vi "Main.vi"(8 "error in (no error)":errorcluster, 11 "ModuleAdmin":refnum<class "ModuleAdmin.lvclass">) -> ()   [LabVIEW 2018, in "DigitizerModule.lvlib"]
uses:
  DigitizerModule.lvlib
  <userlib>/NIST/ModuleAdminLib/ModuleAdmin/ModuleAdmin.lvclass
  C:/Program Files/National Instruments/LabVIEW 2018/user.lib/NIST/ModuleAdminLib/ModuleAdminBase/ModuleAdminBase.lvclass
  PublicAPI/Arguments/Requests/clStopArgument.ctl
  DigitizerPlugins/DigitizerBaseClass/DigitizerBase.lvclass
  C:/Program Files/National Instruments/LabVIEW 2018/user.lib/NIST/BaseClasses/BasePlugin_class/BasePlugin.lvclass
  <userlib>/NIST/ModuleAdminLib/ModuleAdmin/ModuleAdmin.lvclass/ModuleAdmin.ctl
  <userlib>/NIST/BaseClasses/BasePlugin_class/BasePlugin.lvclass/BasePlugin.ctl
  DigitizerPlugins/DigitizerBaseClass/DigitizerBase.lvclass/DigitizerBase.ctl
  DigitizerPlugins/DigitizerBaseClass/Typedefs/Channel.ctl
  DigitizerPlugins/DigitizerBaseClass/Typedefs/Acquisition.ctl
  DigitizerPlugins/DigitizerBaseClass/Typedefs/Trigger.ctl
  DigitizerPlugins/DigitizerBaseClass/Typedefs/TrigSource.ctl
  <vilib>/Utility/error.llb/DialogType.ctl
  <userlib>/NIST/ModuleAdminLib/ModuleAdmin/Accessors/Read ShowPanel_.vi
  <userlib>/NIST/ModuleAdminLib/ModuleAdmin/Accessors/Write ShowPanel_.vi
  <userlib>/NIST/BaseClasses/BasePlugin_class/Accessors/Write PluginIniFilePath.vi
  <userlib>/NIST/BaseClasses/BasePlugin_class/Accessors/Read PluginIniFilePath.vi
  DigitizerPlugins/DigitizerBaseClass/Accessors/Read Channels.vi
  DigitizerPlugins/DigitizerBaseClass/Accessors/Write Channels.vi
  DigitizerPlugins/DigitizerBaseClass/Accessors/Read Acquisition.vi
  DigitizerPlugins/DigitizerBaseClass/Accessors/Write Acquisition.vi
  DigitizerPlugins/DigitizerBaseClass/Accessors/Read Trigger.vi
  DigitizerPlugins/DigitizerBaseClass/Accessors/Write Trigger.vi
  DigitizerPlugins/DigitizerBaseClass/Accessors/Read Waveforms.vi
  <userlib>/NIST/ModuleAdminLib/ModuleAdmin/Accessors/Read CloneRegRef.vi
  <vilib>/Utility/error.llb/Error Cluster From Error Code.vi
  <vilib>/ErrorRing/Error Ring.xnode
  <userlib>/NIST/ModuleAdminLib/CloneRegistration/CloneRegistration.lvclass
  <userlib>/NIST/BaseClasses/Object_class/BaseObject.lvclass
  <userlib>/NIST/ModuleAdminLib/ModuleAdmin.lvlib
panel:
  out "error out":errorcluster
  # "This is the template for your cloneable module.\nYou should modifiy this to perform the functionality\nthat you want it to perform"
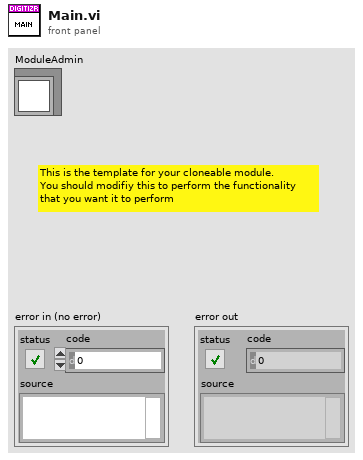
[diagram p1: front panel]
types:
  T1 = typedef "DigitizerModule.lvlib/clRequestEvents.ctl" = cluster{"StopRequest":refnum<user-event>, "PathToINI":refnum<user-event>, " LoadPlugin":refnum<user-event>, "ShowPanel":refnum<user-event>, "PrefDlg":refnum<user-event>, "ReadChannels":refnum<user-event>, "WriteChannels":refnum<user-event>, "ConfigChannels":refnum<user-event>, "ReadAcq":refnum<user-event>, "WriteAcq":refnum<user-event>, "ConfigAcq":refnum<user-event>, "ReadTriggers":refnum<user-event>, "WriteTriggers":refnum<user-event>, "ConfigTriggers":refnum<user-event>, "FetchWfrm":refnum<user-event>, "ReadWfrm":refnum<user-event>, "Initialize":refnum<user-event>, "Abort":refnum<user-event>, "ReadSyncInfo":refnum<user-event>, "WriteSyncInfo":refnum<user-event>}
  T2 = typedef "DigitizerModule.lvlib/clBroadcastEvents.ctl" = cluster{"DidInit":refnum<user-event>, "StatusUpdate":refnum<user-event>, "ErrorReport":refnum<user-event>, "DidStop":refnum<user-event>, "PathToINI":refnum<user-event>, "Channels":refnum<user-event>, "Acq":refnum<user-event>, "Trigger":refnum<user-event>, "Waveforms":refnum<user-event>}
  T3 = typedef "DigitizerModule.lvlib/clStopArgument.ctl" = cluster{"Exit via Stop Module Req?":bool, "Wait for Module to stop?":bool, "ModuleAdmin":refnum<class "ModuleAdmin.lvclass">}
  T4 = enum32{"Invalid", "Standard", "Closed", "Hidden", "Minimized", "Maximized"}
  T5 = typedef "DigitizerPlugins.lvlib/DigitizerBase.lvclass/Channel.ctl" = cluster{"Name":string, "Enabled":bool, "InputImpedance":dbl, "Coupling":enum16{"AC", "DC", "Gnd"}, "Offset":dbl, "Range":dbl}
  T6 = typedef "DigitizerPlugins.lvlib/DigitizerBase.lvclass/Acquisition.ctl" = cluster{"SampleRate":dbl, "RecordSize":i32, "NumRecords":i32, "SampleMode":i32, "Timeout (ms)":i32}
  T7 = typedef "DigitizerPlugins.lvlib/DigitizerBase.lvclass/Trigger.ctl" = cluster{"Source":string, "Delay":dbl, "Holdoff":dbl, "PretriggerSamples":i32, "Sources":T8[]}
  T8 = typedef "DigitizerPlugins.lvlib/DigitizerBase.lvclass/TrigSource.ctl" = cluster{"Name":string, "Coupling":enum16{"AC", "DC", "HF Reject", "LF Reject", "Noise Reject"}, "Hysteresis":dbl, "Level":dbl, "Slope":enum16{"Positive", "Negative"}, "Type":enum16{"Edge", "Width", "Runt", "Glitch", "TV", "Window"}}
  T9 = typedef "DialogType.ctl" = u16
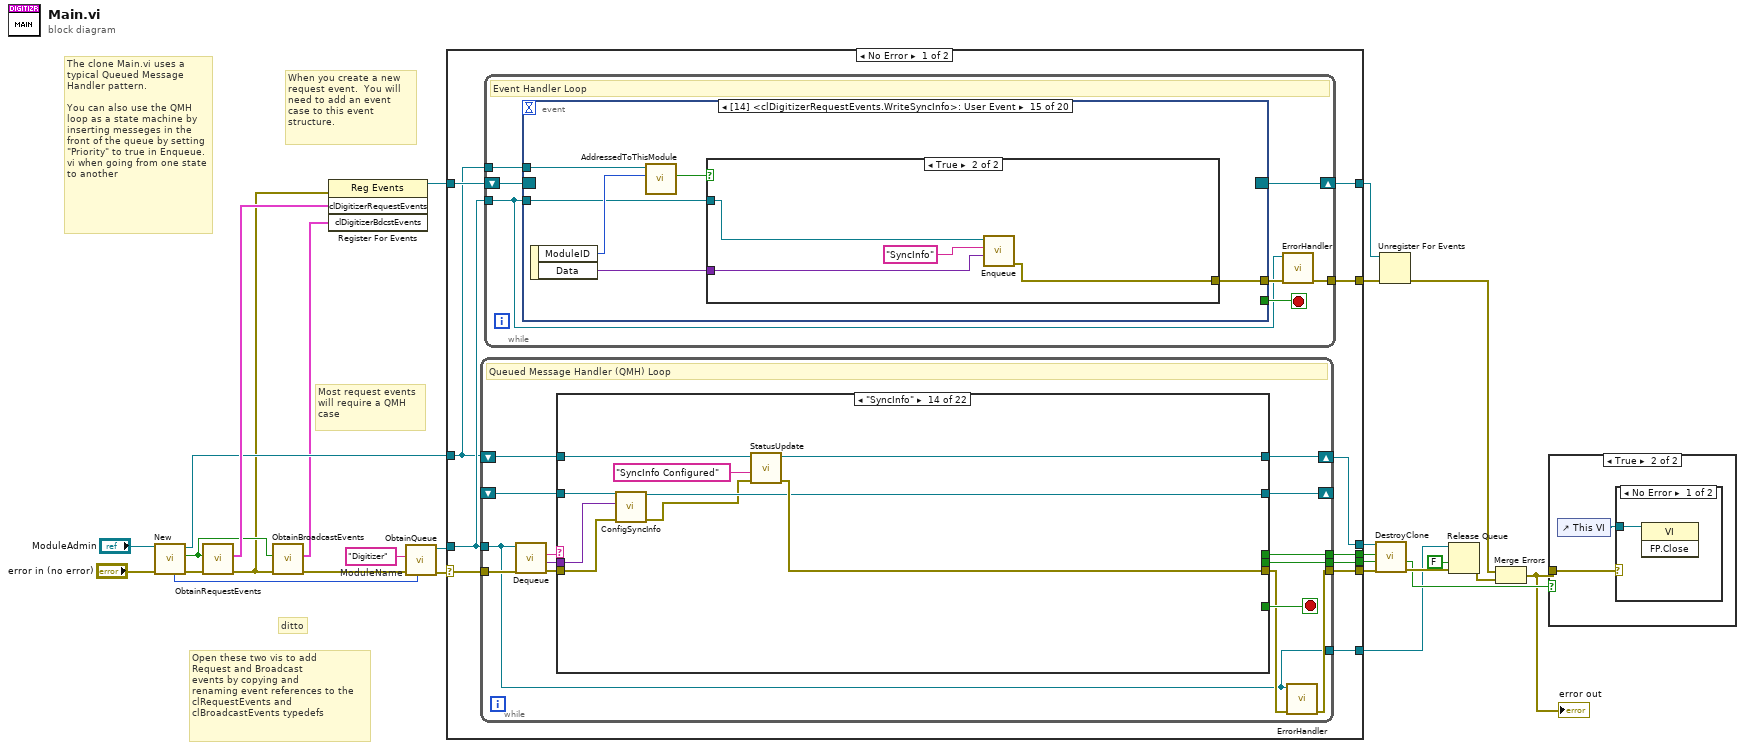
[diagram p0: block diagram]
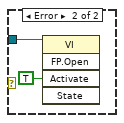
[diagram p3: hidden frame]
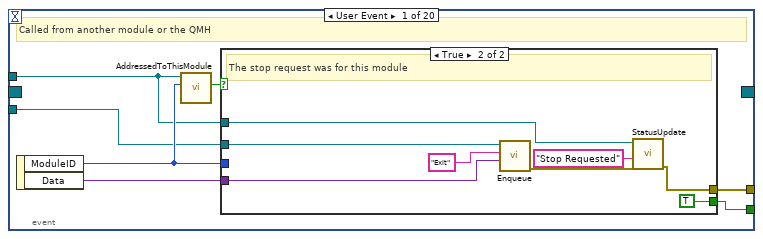
[diagram p4: hidden frame]
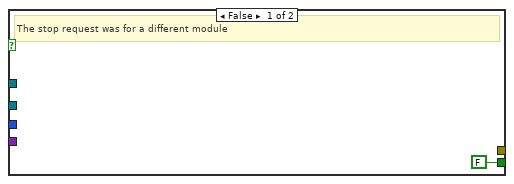
[diagram p5: hidden frame]
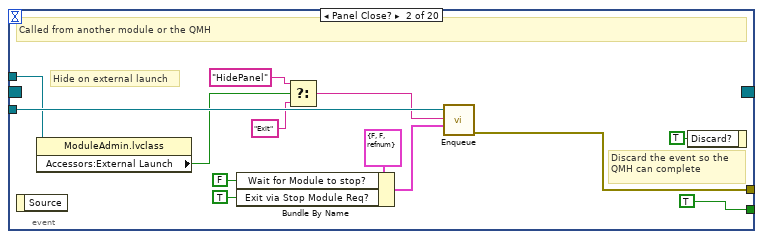
[diagram p6: hidden frame]
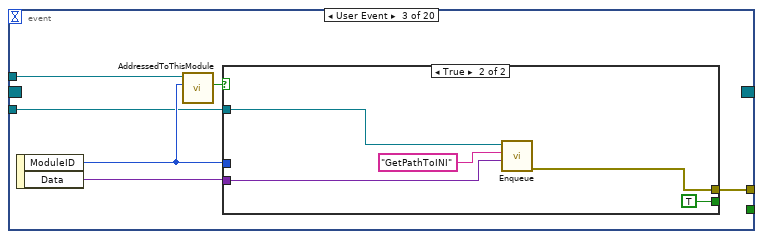
[diagram p7: hidden frame]
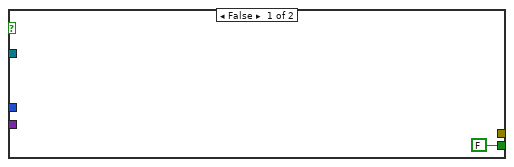
[diagram p8: hidden frame]
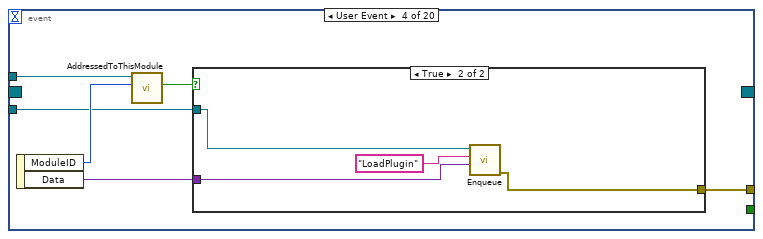
[diagram p9: hidden frame]
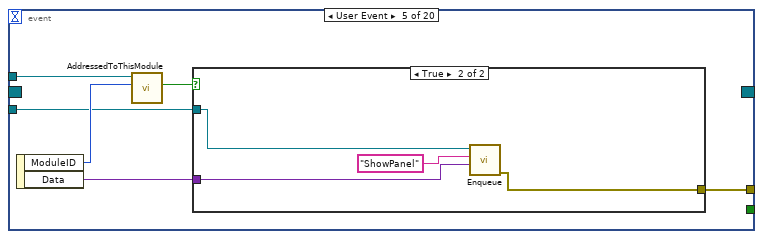
[diagram p11: hidden frame]
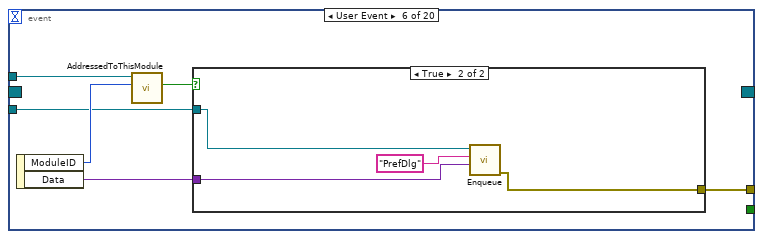
[diagram p13: hidden frame]
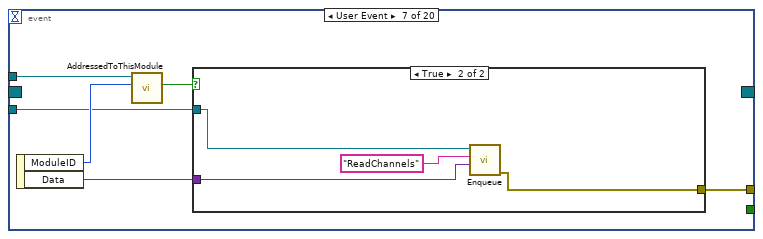
[diagram p15: hidden frame]
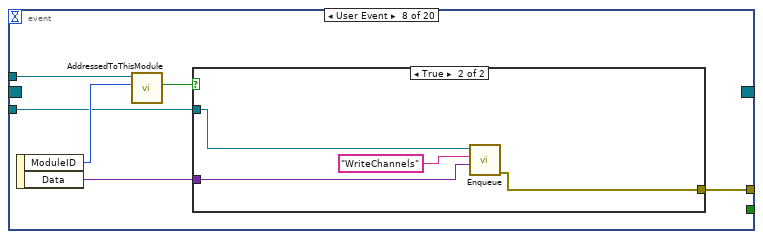
[diagram p17: hidden frame]
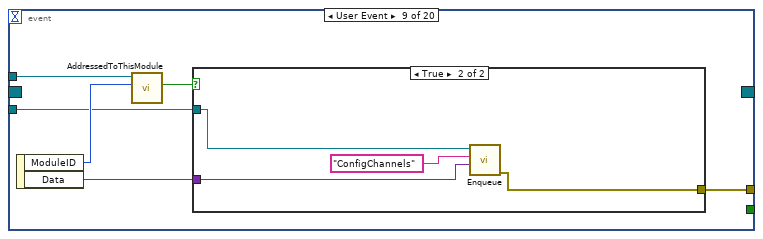
[diagram p19: hidden frame]
diagram:
  w1 = "Digitizer"  # ModuleName
  # "The clone Main.vi uses a typical Queued Message Handler pattern.  \n\nYou can also use the QMH loop as a state machine by inserting messeges in the front of the queue by setting \"Priority\" to true in Enqueue.vi when going from one state to another"
  # "Open these two vis to add\nRequest and Broadcast \nevents by copying and \nrenaming event references to the \nclRequestEvents and \nclBroadcastEvents typedefs"
  # "ditto"
  # "Most request events\nwill require a QMH\ncase"
  # "When you create a new request event.  You will need to add an event case to this event structure."
  n1 = call <userlib>:"New.vi"("error in (no error)"="error in (no error)", "ModuleAdmin"="ModuleAdmin") -> ("error out"=w25:errorcluster, "First?"=w19:bool, "ModuleAdmin"=w21:refnum<class "ModuleAdmin.lvclass">, "Module ID"=w2:i32)  [unwired: 6 in]
  n2 = call "ObtainRequestEvents.vi"("error in (no error)"=w25, "CreateNew (F)"=w19) -> ("error out"=w18:errorcluster, "clDigitizerRequestEvents"=w24:T1)  [unwired: 8 in]
  n3 = call "ObtainBroadcastEvents.vi"("error in (no error)"=w18, "CreateNew? (F)"=w19) -> ("error out"=w20:errorcluster, "clDigitizerBdcstEvents"=w17:T2)  [unwired: 8 in]
  n4 = register-events(error in=w18, w24, w17) -> (reference out=w16:refnum<event-registration>)  [unwired: 1 in, 1 out]
  n5 = call "ObtainQueue.vi"("ModuleID"=w2, "error in (no error)"=w20, "ModuleName"=w1) -> ("error out"=w23:errorcluster, "MessageQueue"=w22:refnum<queue>)  [unwired: 7 in]
  n6 = case shown="No Error" w23 {
    selector: w23 -> [w38 w592]
    tunnel: w22 -> [w36 w584]
    tunnel: w21 -> [w34 w589]
    tunnel: [w37 w590] -> w15
    tunnel: w16 -> [w35 w585]
    tunnel: [w33 w588] -> w13
    tunnel: [w32 _] -> w12
    tunnel: [w31 _] -> w11
    tunnel: [w30 _] -> w8
    tunnel: [w29 w585] -> w7
    tunnel: [w28 w584] -> w4
    frame No Error {
      n7 = while {
        tunnel: w36 -> [w257]
        tunnel: w38 -> [w269]
        tunnel: [w262] -> w37
        tunnel: [w264] -> w32
        tunnel: [w263] -> w31
        shift-right: [w260] -> _
        shift-left: _ -> [w259]
        shift-right: [w258] -> w33
        shift-left: w34 -> [w265]
        tunnel: [w257] -> w28
        stop <- w270 stop-if-true
        # "Queued Message Handler (QMH) Loop"
        n8 = call "Dequeue.vi"("error in (no error)"=w269, "MessageQueue"=w257) -> ("error out"=w268:errorcluster, "Message Data"=w266:variant, "Message"=w267:string)  [unwired: 6 in, 1 out]
        n9 = case shown="\"SyncInfo\"" w267 {
          selector: w267 -> [_ _ _ _ _ _ _ _ _ _ _ _ _ _ _ _ _ _ _ _ _ w572]
          tunnel: [_ _ _ _ _ _ _ _ _ _ _ _ _ _ _ _ _ _ _ TRUE _ _] -> w270
          tunnel: w265 -> [w291 w308 w316 w363 w366 w377 w382 w397 w411 w416 w431 w445 w450 w467 w474 w485 w505 w520 w531 w543 w553 w575]
          tunnel: [w280 w301 w317 w364 w369 w371 w379 w391 w406 w413 w425 w440 w447 w464 w468 w483 w496 w512 w527 w549 w554 w571] -> w261
          tunnel: w268 -> [_ w311 w326 w359 w370 w375 w389 w394 w410 w423 w426 w444 w457 w461 w471 w487 w503 w517 w530 w540 w562 _]
          tunnel: w266 -> [_ w310 w328 _ _ _ w390 _ _ w424 _ _ w458 w462 _ _ _ _ _ w548 w561 _]
          tunnel: [_ _ _ _ _ _ _ _ _ _ _ _ _ _ _ _ _ _ _ w546 _ _] -> w264
          tunnel: [_ _ _ _ _ _ _ _ _ _ _ _ _ _ _ _ _ _ _ w545 _ _] -> w263
          tunnel: [refnum<class "DigitizerBase.lvclass"> refnum ("MyPlugins.lvlib:MyPluginsBase.lvclass") w300 w314 w360 w367 w373 w385 w392 w408 w419 w428 w442 w453 w460 w469 w484 w498 w515 w528 w544 w552 w569] -> w260
          tunnel: w259 -> [_ w300 w315 w362 w368 w378 w387 w395 w412 w421 w429 w446 w455 w463 w472 w488 w501 w519 w529 w544 w552 w569]
          tunnel: [w271 w307 w312 w357 w366 w372 w381 w396 w407 w415 w430 w441 w449 w466 w473 w482 w497 w513 w532 w542 w551 w568] -> w258
          frame "Initialize" {
            # "Initialize is always called after ObtainQueue.vi is run"
            n10 = property class="ModuleAdmin.lvclass"(reference=w291) -> (reference out=w277:refnum<class "ModuleAdmin.lvclass">, error out=w288:errorcluster, "Accessors:Module ID"=w279:i32, "Accessors:ShowPanel_"=w274:bool, "Accessors:External Launch"=w273:bool, "Accessors:ModuleName"=w275:string)  [unwired: 1 in]
            n11 = Compound Arithmetic op=OR(w274, invert w273) -> (w272:bool)
            n12 = Select(t=T4."Standard" ("Front Panel Window:State"), s=w272, f=T4."Hidden" ("Front Panel Window:State")) -> (s? t:f=w284:T4)
            n13 = invoke class="VI" method="FP.Open"(error in=w288, "State"=w284) -> (error out=w287:errorcluster)  [unwired: 3 in, 4 out]
            n14 = call <userlib>:"ModuleName.vi"("Name"=w275, "ModuleID"=w279) -> ("ModuleName"=w283:string)  [unwired: 9 in]
            n15 = property class="VI"(error in=w287, "Front Panel.Title"=w283) -> (reference out=w290:refnum<vi>, error out=w289:errorcluster)  [unwired: 1 in]
            n16 = invoke class="VI" method="FP.Center"(reference=w290, error in=w289) -> (error out=w278:errorcluster)  [unwired: 1 in, 2 out]
            n17 = case shown="True" w273 {
              tunnel: [w292 w298] -> w281
              tunnel: [w293 w295] -> w271
              tunnel: w278 -> [w292 w297]
              tunnel: w277 -> [w293 w294]
              frame False {
              }
              frame True {
                n18 = call <userlib>:"WaitOnModuleSync.vi"("error in (no error)"=w297, "ModuleAdmin"=w294) -> ("error out"=w299:errorcluster, "ModuleAdmin"=w296:refnum<class "ModuleAdmin.lvclass">)  [unwired: 8 in]
                n19 = call <userlib>:"WaitOnEventSync.vi"("error in (no error)"=w299, "ModuleAdmin"=w296) -> ("error out"=w298:errorcluster, "ModuleAdmin"=w295:refnum<class "ModuleAdmin.lvclass">)  [unwired: 8 in]
              }
            }
            n20 = call "DidInit.vi"("Init?"=TRUE, "error in (no error)"=w281, "ModuleAdmin"=w271) -> ("error out"=w280:errorcluster)  [unwired: 8 in]
          }
          frame "ShowPanel" {
            # "The frontpanel can be shown or hidden"
            n21 = Variant To Data(error in=w311, type=TRUE, Variant=w310) -> (data=w303:bool, error out=w306:errorcluster)
            n22 = Select(t=T4."Standard" ("Front Panel Window:State"), s=w303, f=T4."Hidden" ("Front Panel Window:State")) -> (s? t:f=w302:T4)
            n23 = property class="VI"(error in=w306, "FP.State"=w302) -> (error out=w301:errorcluster)  [unwired: 1 in, 1 out]
            n24 = property class="ModuleAdmin.lvclass"(reference=w308, "Accessors:ShowPanel_"=w303) -> (reference out=w307:refnum<class "ModuleAdmin.lvclass">)  [unwired: 1 in, 1 out]
          }
          frame "LoadPlugin" {
            # "Dynamically oads and initializes a plugin from the .ini file"
            n25 = Variant To Data(error in=w326, type=path "", Variant=w328) -> (data=w313:path, error out=w325:errorcluster)
            n26 = call <userlib>:"GetPathToClass.vi"("error in (no error)"=w325, "configuration file path"=w313) -> ("error IO"=w321:errorcluster, "PathToClass"=w324:path)  [unwired: 8 in]
            n27 = Current VI's Path() -> (path=w323:path)
            n28 = Build Path(base path=w323, name or relative path=w324) -> (appended path=w322:path)
            n29 = call <vilib>:"Check if File or Folder Exists.vi"("error in (no error)"=w321, "path"=w322) -> ("error out"=w318:errorcluster, "file or folder exists?"=w320:bool, "dup path"=w319:path)  [unwired: 7 in]
            n30 = case shown="True" w320 {
              tunnel: w319 -> [w332 w349]
              tunnel: w318 -> [_ w356]
              tunnel: [w331 w351] -> w317
              tunnel: w316 -> [w329 w346]
              tunnel: w315 -> [w330 _]
              tunnel: [w330 w342] -> w314
              tunnel: w313 -> [_ w347]
              tunnel: [w329 w345] -> w312
              frame False {
                n31 = Path To String(path=w332) -> (string=w333:string)
                n32 = xnode "Error Ring"("parameter 0"=w333) -> ("error out"=w331:errorcluster)
              }
              frame True {
                n33 = call-dynamic "LoadClassFromFile.vi"("error in (no error)"=w356, "class path"=w349, "reference in"=refnum<class "DigitizerBase.lvclass"> refnum ("MyPlugins.lvlib:MyPluginsBase.lvclass")) -> ("error out"=w348:errorcluster, "reference out"=w350:refnum<class "DigitizerBase.lvclass">)  [unwired: 7 in]
                n34 = property class="DigitizerBase.lvclass"(reference=w350, error in=w348, "Accessors:PluginIniFilePath"=w347) -> (reference out=w344:refnum<class "DigitizerBase.lvclass">, error out=w343:errorcluster)
                n35 = Path To String(path=w349) -> (string=w353:string)
                n36 = Format Into String(format string="Plugin %s loaded ", w353) -> (resulting string=w352:string)  [unwired: 2 in, 1 out]
                n37 = call-dynamic "DefaultFromIni.vi"("error in (no error)"=w343, "MyPluginsBase in"=w344) -> ("error out"=w341:errorcluster, "MyPluginsBase out"=w342:refnum<class "DigitizerBase.lvclass">)  [unwired: 8 in]
                n38 = call "StatusUpdate.vi"("error in (no error)"=w341, "Status"=w352, "Module"=w346) -> ("error out"=w351:errorcluster, "Module"=w345:refnum<class "ModuleAdmin.lvclass">)  [unwired: 7 in]
              }
            }
          }
          frame "GetPathToINI" {
            # "Broadcast the path to the .ini file"
            n39 = property class="DigitizerBase.lvclass"(reference=w362, error in=w359) -> (reference out=w360:refnum<class "DigitizerBase.lvclass">, error out=w358:errorcluster, "Accessors:PluginIniFilePath"=w361:path)
            n40 = property class="ModuleAdmin.lvclass"(reference=w363) -> (reference out=w357:refnum<class "ModuleAdmin.lvclass">, "Accessors:Module ID"=w365:i32)  [unwired: 1 in, 1 out]
            n41 = call "PathToINIBroadcast.vi"("error in (no error)"=w358, "PathToINI"=w361, "ModuleID"=w365) -> ("error out"=w364:errorcluster)  [unwired: 8 in]
          }
          frame "PrefDlg" {
            # "Override Base Class\\PublicMethods\\PrefDialog.vi for user editable preference dialog"
            # "Launch the modal Preferences dialog"
            n42 = call-dynamic "PrefDialog.vi"("error in (no error)"=w370, "MyPluginsBase in"=w368) -> ("error out"=w369:errorcluster, "MyPluginsBase out"=w367:refnum<class "DigitizerBase.lvclass">)  [unwired: 8 in]
          }
          frame "ReadChannels" {
            n43 = property class="DigitizerBase.lvclass"(reference=w378, error in=w375) -> (reference out=w373:refnum<class "DigitizerBase.lvclass">, error out=w374:errorcluster, "Accessors:Channels"=w376:T5[])
            n44 = call "ChannelBdcst.vi"("error in (no error)"=w374, "Channels"=w376, "Module"=w377) -> ("error out"=w371:errorcluster, "Module"=w372:refnum<class "ModuleAdmin.lvclass">)  [unwired: 7 in]
          }
          frame "WriteChannels" {
            n45 = Variant To Data(error in=w389, type=T5[] [], Variant=w390) -> (data=w386:T5[], error out=w384:errorcluster)
            n46 = property class="DigitizerBase.lvclass"(reference=w387, error in=w384, "Accessors:Channels"=w386) -> (reference out=w385:refnum<class "DigitizerBase.lvclass">, error out=w383:errorcluster)
            n47 = call "StatusUpdate.vi"("error in (no error)"=w383, "Status"="Received Channels", "Module"=w382) -> ("error out"=w379:errorcluster, "Module"=w381:refnum<class "ModuleAdmin.lvclass">)  [unwired: 7 in]
          }
          frame "ConfigChannels" {
            n48 = call-dynamic "ConfigChannels.vi"("error in (no error)"=w394, "DigitizerBase in"=w395) -> ("error out"=w393:errorcluster, "DigitizerBase out"=w392:refnum<class "DigitizerBase.lvclass">)  [unwired: 8 in]
            n49 = case shown="No Error" w393 {
              selector: w393 -> [w402 w403]
              tunnel: w397 -> [w401 w404]
              tunnel: [w399 w403] -> w391
              tunnel: [w398 w404] -> w396
              frame No Error {
                n50 = call "StatusUpdate.vi"("error in (no error)"=w402, "Status"="Channels Configured", "Module"=w401) -> ("error out"=w399:errorcluster, "Module"=w398:refnum<class "ModuleAdmin.lvclass">)  [unwired: 7 in]
              }
              frame Error {
              }
            }
          }
          frame "ReadAcq" {
            n51 = property class="DigitizerBase.lvclass"(reference=w412, error in=w410) -> (reference out=w408:refnum<class "DigitizerBase.lvclass">, error out=w409:errorcluster, "Accessors:Acquisition"=w405:T6)
            n52 = call "AcqBdcst.vi"("error in (no error)"=w409, "Acquisition"=w405, "Module"=w411) -> ("error out"=w406:errorcluster, "Module"=w407:refnum<class "ModuleAdmin.lvclass">)  [unwired: 7 in]
          }
          frame "WriteAcq" {
            n53 = Variant To Data(error in=w423, type=T6 {"SampleRate"=0.0, "RecordSize"=0, "NumRecords"=0, "SampleMode"=0, "Timeout (ms)"=0}, Variant=w424) -> (data=w420:T6, error out=w418:errorcluster)
            n54 = property class="DigitizerBase.lvclass"(reference=w421, error in=w418, "Accessors:Acquisition"=w420) -> (reference out=w419:refnum<class "DigitizerBase.lvclass">, error out=w417:errorcluster)
            n55 = call "StatusUpdate.vi"("error in (no error)"=w417, "Status"="Received Acquisition", "Module"=w416) -> ("error out"=w413:errorcluster, "Module"=w415:refnum<class "ModuleAdmin.lvclass">)  [unwired: 7 in]
          }
          frame "ConfigAcq" {
            n56 = call-dynamic "ConfigAcq.vi"("error in (no error)"=w426, "DigitizerBase in"=w429) -> ("error out"=w427:errorcluster, "DigitizerBase out"=w428:refnum<class "DigitizerBase.lvclass">)  [unwired: 8 in]
            n57 = case shown="No Error" w427 {
              selector: w427 -> [w436 w437]
              tunnel: w431 -> [w435 w438]
              tunnel: [w433 w437] -> w425
              tunnel: [w432 w438] -> w430
              frame No Error {
                n58 = call "StatusUpdate.vi"("error in (no error)"=w436, "Status"="Acquisition Configured", "Module"=w435) -> ("error out"=w433:errorcluster, "Module"=w432:refnum<class "ModuleAdmin.lvclass">)  [unwired: 7 in]
              }
              frame Error {
              }
            }
          }
          frame "ReadTriggers" {
            n59 = property class="DigitizerBase.lvclass"(reference=w446, error in=w444) -> (reference out=w442:refnum<class "DigitizerBase.lvclass">, error out=w443:errorcluster, "Accessors:Trigger"=w439:T7)
            n60 = call "TriggerBdcst.vi"("error in (no error)"=w443, "Trigger"=w439, "Module"=w445) -> ("error out"=w440:errorcluster, "Module"=w441:refnum<class "ModuleAdmin.lvclass">)  [unwired: 7 in]
          }
          frame "WriteTrigger" {
            n61 = Variant To Data(error in=w457, type=T7 {"Source"="", "Delay"=0.0, "Holdoff"=0.0, "PretriggerSamples"=0, "Sources"=[]}, Variant=w458) -> (data=w454:T7, error out=w452:errorcluster)
            n62 = property class="DigitizerBase.lvclass"(reference=w455, error in=w452, "Accessors:Trigger"=w454) -> (reference out=w453:refnum<class "DigitizerBase.lvclass">, error out=w451:errorcluster)
            n63 = call "StatusUpdate.vi"("error in (no error)"=w451, "Status"="Received Trigger", "Module"=w450) -> ("error out"=w447:errorcluster, "Module"=w449:refnum<class "ModuleAdmin.lvclass">)  [unwired: 7 in]
          }
          frame "SyncInfo" {
            n64 = call-dynamic "ConfigSyncInfo.vi"("error in (no error)"=w461, "SyncInfo"=w462, "DigitizerBase in"=w463) -> ("error out"=w459:errorcluster, "DigitizerBase out"=w460:refnum<class "DigitizerBase.lvclass">)  [unwired: 7 in]
            n65 = call "StatusUpdate.vi"("error in (no error)"=w459, "Status"="SyncInfo Configured", "Module"=w467) -> ("error out"=w464:errorcluster, "Module"=w466:refnum<class "ModuleAdmin.lvclass">)  [unwired: 7 in]
          }
          frame "ConfigTrigger" {
            n66 = call-dynamic "ConfigTrigger.vi"("error in (no error)"=w471, "DigitizerBase in"=w472) -> ("error out"=w470:errorcluster, "DigitizerBase out"=w469:refnum<class "DigitizerBase.lvclass">)  [unwired: 8 in]
            n67 = case shown="No Error" w470 {
              selector: w470 -> [w479 w480]
              tunnel: w474 -> [w478 w481]
              tunnel: [w476 w480] -> w468
              tunnel: [w475 w481] -> w473
              frame No Error {
                n68 = call "StatusUpdate.vi"("error in (no error)"=w479, "Status"="Trigger Configured", "Module"=w478) -> ("error out"=w476:errorcluster, "Module"=w475:refnum<class "ModuleAdmin.lvclass">)  [unwired: 7 in]
              }
              frame Error {
              }
            }
          }
          frame "InitDevice" {
            n69 = call-dynamic "Initialize.vi"("error in (no error)"=w487, "DigitizerBase in"=w488) -> ("error out"=w486:errorcluster, "DigitizerBase out"=w484:refnum<class "DigitizerBase.lvclass">)  [unwired: 8 in]
            n70 = case shown="No Error" w486 {
              selector: w486 -> [w493 w494]
              tunnel: w485 -> [w492 w495]
              tunnel: [w490 w494] -> w483
              tunnel: [w489 w495] -> w482
              frame No Error {
                n71 = call "StatusUpdate.vi"("error in (no error)"=w493, "Status"="Digitizer Initialized", "Module"=w492) -> ("error out"=w490:errorcluster, "Module"=w489:refnum<class "ModuleAdmin.lvclass">)  [unwired: 7 in]
              }
              frame Error {
              }
            }
          }
          frame "FetchWfrms" {
            n72 = call "StatusUpdate.vi"("error in (no error)"=w503, "Status"="Beginning Fetch", "Module"=w505) -> ("error out"=w502:errorcluster, "Module"=w499:refnum<class "ModuleAdmin.lvclass">)  [unwired: 7 in]
            n73 = call-dynamic "FetchAllDbl.vi"("error in (no error)"=w502, "DigitizerBase in"=w501) -> ("error out"=w500:errorcluster, "DigitizerBase out"=w498:refnum<class "DigitizerBase.lvclass">)  [unwired: 8 in]
            n74 = case shown="No Error" w500 {
              selector: w500 -> [_ w510]
              tunnel: w499 -> [w509 w511]
              tunnel: [w507 w511] -> w497
              tunnel: [w506 w510] -> w496
              frame No Error {
                n75 = call "StatusUpdate.vi"("Status"="Fetch Complete", "Module"=w509) -> ("error out"=w506:errorcluster, "Module"=w507:refnum<class "ModuleAdmin.lvclass">)  [unwired: 8 in]
              }
              frame Error {
              }
            }
          }
          frame "ReadWfrms" {
            n76 = property class="DigitizerBase.lvclass"(reference=w519, error in=w517) -> (reference out=w515:refnum<class "DigitizerBase.lvclass">, error out=w516:errorcluster, "Accessors:Waveforms"=w518:variant)
            n77 = call "WfrmBdcst.vi"("error in (no error)"=w516, "Waveforms"=w518, "Module"=w520) -> ("error out"=w512:errorcluster, "Module"=w514:refnum<class "ModuleAdmin.lvclass">)  [unwired: 7 in]
            n78 = case shown="No Error" w512 {
              selector: w512 -> [_ w525]
              tunnel: w514 -> [w524 w526]
              tunnel: [w522 w526] -> w513
              tunnel: [w521 w525] -> _
              frame No Error {
                n79 = call "StatusUpdate.vi"("Status"="Read Complete", "Module"=w524) -> ("error out"=w521:errorcluster, "Module"=w522:refnum<class "ModuleAdmin.lvclass">)  [unwired: 8 in]
              }
              frame Error {
              }
            }
          }
          frame "Abort" {
            n80 = call-dynamic "Abort.vi"("error in (no error)"=w530, "DigitizerBase in"=w529) -> ("error out"=w527:errorcluster, "DigitizerBase out"=w528:refnum<class "DigitizerBase.lvclass">)  [unwired: 8 in]
            n81 = case shown="No Error" w527 {
              selector: w527 -> [_ w537]
              tunnel: w531 -> [w536 w538]
              tunnel: [w534 w538] -> w532
              tunnel: [w533 w537] -> _
              frame No Error {
                n82 = call "StatusUpdate.vi"("Status"="Abort Complete", "Module"=w536) -> ("error out"=w533:errorcluster, "Module"=w534:refnum<class "ModuleAdmin.lvclass">)  [unwired: 8 in]
              }
              frame Error {
              }
            }
          }
          frame "Exit" {
            # "Called by the StopRequest event handler case"
            n83 = call "StatusUpdate.vi"("error in (no error)"=w540, "Status"="Exiting", "Module"=w543) -> ("error out"=w539:errorcluster, "Module"=w542:refnum<class "ModuleAdmin.lvclass">)  [unwired: 7 in]
            n84 = control-ref of="This VI"() -> (w547:refnum<vi>)
            n85 = call "HandleExit.vi"("error in (no error)"=w539, "VI Refnum"=w547, "StopArgument"=w548, "ModuleAdmin"=w542) -> ("error out"=w549:errorcluster, "Exit via Stop Module Req?"=w545:bool, "WaitForStop?"=w546:bool)  [unwired: 5 in]
          }
          frame "Error" {
            # "Handle any errors"
            n86 = property class="ModuleAdmin.lvclass"(reference=w553) -> (reference out=w551:refnum<class "ModuleAdmin.lvclass">, "Accessors:External Launch"=w557:bool, "Accessors:Module ID"=w555:i32)  [unwired: 1 in, 1 out]
            n87 = Variant To Data(error in=w562, type=errorcluster {"status"=FALSE, "code"=0, "source"=""} ("error constant"), Variant=w561) -> (data=w556:errorcluster, error out=w559:errorcluster)
            n88 = call "ReportError.vi"("error in (no error)"=w559, "ErrorReported"=w556, "ModuleID"=w555) -> ("error out"=w558:errorcluster)  [unwired: 8 in]
            n89 = case shown="True" w557 {
              tunnel: w558 -> [w566 w567]
              tunnel: w556 -> [w565 _]
              tunnel: [w564 w567] -> w554
              tunnel: w553 -> [w563 _]
              frame False {
                # "Todo:  Add an event to ask the user\nIf the module should stop or continue"
                # "Stand alone: now, force an exit"
                n90 = call <vilib>:"Simple Error Handler.vi"("error in (no error)"=w565) -> ()  [unwired: 4 in, 5 out]
                n91 = call "StopRequest.vi"("error in (no error)"=w566, "ModuleAdmin"=w563) -> ("error out"=w564:errorcluster)  [unwired: 8 in, 1 out]
              }
              frame True {
                # "Externally launched modules only broadcast the error msg"
              }
            }
          }
          frame Default {
            # "Called only if a message was queued and no QMH case was created"
            n92 = property class="ModuleAdmin.lvclass"(reference=w575) -> (reference out=w568:refnum<class "ModuleAdmin.lvclass">, "Accessors:Module ID"=w574:i32, "Accessors:ModuleName"=w570:string)  [unwired: 1 in, 1 out]
            n93 = call <userlib>:"ModuleName.vi"("Name"=w570, "ModuleID"=w574) -> ("ModuleName"=w573:string)  [unwired: 9 in]
            n94 = xnode "Error Ring"("parameter 0"=w572, "parameter 1"=w573) -> ("error out"=w571:errorcluster)
          }
        }
        n95 = call "ErrorHandler.vi"("error in (no error)"=w261, "MessageQueue"=w257) -> ("error out"=w262:errorcluster)  [unwired: 8 in, 1 out]
      }
      n96 = while {
        tunnel: w36 -> [w39]
        shift-right: [w43] -> w29
        shift-left: w35 -> [w44]
        tunnel: w34 -> [w42]
        tunnel: [w40] -> w30
        stop <- w45 stop-if-true
        # "Event Handler Loop"
        n97 = event shown="[14] <clDigitizerRequestEvents.WriteSyncInfo>: User Event" {
          selector: w44 -> [_ _ _ _ _ _ _ _ _ _ _ _ _ _ _ _ _ _ _ _]
          dyn-events: [_ _ _ _ _ _ _ _ _ _ _ _ _ _ _ _ _ _ _ _] -> w43
          timeout: _ -> [_ _ _ _ _ _ _ _ _ _ _ _ _ _ _ _ _ _ _ _]
          tunnel: w39 -> [w50 w74 w77 w88 w98 w108 w118 w128 w138 w148 w158 w168 w178 w188 w198 w208 w218 w228 w238 w248]
          tunnel: [w49 TRUE _ _ _ _ _ _ _ _ _ _ _ _ _ _ _ _ _ _] -> w45
          tunnel: w42 -> [w46 w68 w76 w92 w102 w112 w122 w132 w142 w152 w162 w172 w182 w192 w202 w212 w222 w232 w242 w252]
          tunnel: [w48 w72 w75 w89 w99 w109 w119 w129 w139 w149 w159 w169 w179 w189 w199 w209 w219 w229 w239 w249] -> w41
          event User Event {
            # "Called from another module or the QMH"
            n98 = event-data() -> ("ModuleID"=w51:i32, "Data"=w47:variant)  [unwired: 1 in]
            n99 = call <userlib>:"AddressedToThisModule.vi"("ModuleID"=w51, "ModuleAdmin"=w46) -> ("AddressedToThisInstance?"=w52:bool)  [unwired: 8 in, 1 out]
            n100 = case shown="True" w52 {
              tunnel: w51 -> [_ _]
              tunnel: w50 -> [_ w61]
              tunnel: [FALSE TRUE] -> w49
              tunnel: [_ w56] -> w48
              tunnel: w47 -> [_ w58]
              tunnel: w46 -> [_ w54]
              frame False {
                # "The stop request was for a different module"
              }
              frame True {
                # "The stop request was for this module"
                n101 = call "Enqueue.vi"("Message Data"=w58, "Message"="Exit", "MessageQueue"=w61) -> ("error out"=w57:errorcluster)  [unwired: 7 in, 1 out]
                n102 = call "StatusUpdate.vi"("error in (no error)"=w57, "Status"="Stop Requested", "Module"=w54) -> ("error out"=w56:errorcluster)  [unwired: 7 in, 1 out]
              }
            }
          }
          event Panel Close? {
            # "Hide on external launch"
            # "Discard the event so the QMH can complete"
            # "Called from another module or the QMH"
            n103 = event-data() -> ()  [unwired: 1 in, 1 out]
            n104 = property class="ModuleAdmin.lvclass"(reference=w68) -> ("Accessors:External Launch"=w63:bool)  [unwired: 1 in, 2 out]
            n105 = Bundle By Name(cluster=T3 {"Exit via Stop Module Req?"=FALSE, "Wait for Module to stop?"=FALSE, "ModuleAdmin"=refnum} ("Stop Argument"), "Wait for Module to stop?"=FALSE, "Exit via Stop Module Req?"=TRUE) -> (w69:T3)
            n106 = Select(t="HidePanel", s=w63, f="Exit" ("Message")) -> (s? t:f=w65:string)
            n107 = call "Enqueue.vi"("Message Data"=w69, "Message"=w65, "MessageQueue"=w74) -> ("error out"=w72:errorcluster)  [unwired: 7 in, 1 out]
            n108 = event-data("Discard?"=TRUE) -> ()  [unwired: 1 in, 1 out]
          }
          event User Event {
            n109 = event-data() -> ("ModuleID"=w78:i32, "Data"=w79:variant)  [unwired: 1 in]
            n110 = call <userlib>:"AddressedToThisModule.vi"("ModuleID"=w78, "ModuleAdmin"=w76) -> ("AddressedToThisInstance?"=w80:bool)  [unwired: 8 in, 1 out]
            n111 = case shown="True" w80 {
              tunnel: w78 -> [_ _]
              tunnel: w77 -> [_ w86]
              tunnel: [FALSE TRUE] -> _
              tunnel: [_ w84] -> w75
              tunnel: w79 -> [_ w82]
              frame False {
                # "The stop request was for a different module"
              }
              frame True {
                # "The stop request was for this module"
                n112 = call "Enqueue.vi"("Message Data"=w82, "Message"="GetPathToINI", "MessageQueue"=w86) -> ("error out"=w84:errorcluster)  [unwired: 7 in, 1 out]
              }
            }
          }
          event User Event {
            n113 = event-data() -> ("ModuleID"=w91:i32, "Data"=w87:variant)  [unwired: 1 in]
            n114 = call <userlib>:"AddressedToThisModule.vi"("ModuleID"=w91, "ModuleAdmin"=w92) -> ("AddressedToThisInstance?"=w90:bool)  [unwired: 8 in, 1 out]
            n115 = case shown="True" w90 {
              tunnel: [_ w93] -> w89
              tunnel: w88 -> [_ w96]
              tunnel: w87 -> [_ w94]
              frame False {
              }
              frame True {
                n116 = call "Enqueue.vi"("Message Data"=w94, "Message"="LoadPlugin", "MessageQueue"=w96) -> ("error out"=w93:errorcluster)  [unwired: 7 in, 1 out]
              }
            }
          }
          event User Event {
            n117 = event-data() -> ("ModuleID"=w101:i32, "Data"=w97:variant)  [unwired: 1 in]
            n118 = call <userlib>:"AddressedToThisModule.vi"("ModuleID"=w101, "ModuleAdmin"=w102) -> ("AddressedToThisInstance?"=w100:bool)  [unwired: 8 in, 1 out]
            n119 = case shown="True" w100 {
              tunnel: [_ w103] -> w99
              tunnel: w98 -> [_ w106]
              tunnel: w97 -> [_ w104]
              frame False {
              }
              frame True {
                n120 = call "Enqueue.vi"("Message Data"=w104, "Message"="ShowPanel", "MessageQueue"=w106) -> ("error out"=w103:errorcluster)  [unwired: 7 in, 1 out]
              }
            }
          }
          event User Event {
            n121 = event-data() -> ("ModuleID"=w111:i32, "Data"=w107:variant)  [unwired: 1 in]
            n122 = call <userlib>:"AddressedToThisModule.vi"("ModuleID"=w111, "ModuleAdmin"=w112) -> ("AddressedToThisInstance?"=w110:bool)  [unwired: 8 in, 1 out]
            n123 = case shown="True" w110 {
              tunnel: [_ w113] -> w109
              tunnel: w108 -> [_ w116]
              tunnel: w107 -> [_ w114]
              frame False {
              }
              frame True {
                n124 = call "Enqueue.vi"("Message Data"=w114, "Message"="PrefDlg", "MessageQueue"=w116) -> ("error out"=w113:errorcluster)  [unwired: 7 in, 1 out]
              }
            }
          }
          event User Event {
            n125 = event-data() -> ("ModuleID"=w121:i32, "Data"=w117:variant)  [unwired: 1 in]
            n126 = call <userlib>:"AddressedToThisModule.vi"("ModuleID"=w121, "ModuleAdmin"=w122) -> ("AddressedToThisInstance?"=w120:bool)  [unwired: 8 in, 1 out]
            n127 = case shown="True" w120 {
              tunnel: [_ w123] -> w119
              tunnel: w118 -> [_ w126]
              tunnel: w117 -> [_ w124]
              frame False {
              }
              frame True {
                n128 = call "Enqueue.vi"("Message Data"=w124, "Message"="ReadChannels", "MessageQueue"=w126) -> ("error out"=w123:errorcluster)  [unwired: 7 in, 1 out]
              }
            }
          }
          event User Event {
            n129 = event-data() -> ("ModuleID"=w131:i32, "Data"=w127:variant)  [unwired: 1 in]
            n130 = call <userlib>:"AddressedToThisModule.vi"("ModuleID"=w131, "ModuleAdmin"=w132) -> ("AddressedToThisInstance?"=w130:bool)  [unwired: 8 in, 1 out]
            n131 = case shown="True" w130 {
              tunnel: [_ w133] -> w129
              tunnel: w128 -> [_ w136]
              tunnel: w127 -> [_ w134]
              frame False {
              }
              frame True {
                n132 = call "Enqueue.vi"("Message Data"=w134, "Message"="WriteChannels", "MessageQueue"=w136) -> ("error out"=w133:errorcluster)  [unwired: 7 in, 1 out]
              }
            }
          }
          event User Event {
            n133 = event-data() -> ("ModuleID"=w141:i32, "Data"=w137:variant)  [unwired: 1 in]
            n134 = call <userlib>:"AddressedToThisModule.vi"("ModuleID"=w141, "ModuleAdmin"=w142) -> ("AddressedToThisInstance?"=w140:bool)  [unwired: 8 in, 1 out]
            n135 = case shown="True" w140 {
              tunnel: [_ w143] -> w139
              tunnel: w138 -> [_ w146]
              tunnel: w137 -> [_ w144]
              frame False {
              }
              frame True {
                n136 = call "Enqueue.vi"("Message Data"=w144, "Message"="ConfigChannels", "MessageQueue"=w146) -> ("error out"=w143:errorcluster)  [unwired: 7 in, 1 out]
              }
            }
          }
          event User Event {
            n137 = event-data() -> ("ModuleID"=w151:i32, "Data"=w147:variant)  [unwired: 1 in]
            n138 = call <userlib>:"AddressedToThisModule.vi"("ModuleID"=w151, "ModuleAdmin"=w152) -> ("AddressedToThisInstance?"=w150:bool)  [unwired: 8 in, 1 out]
            n139 = case shown="True" w150 {
              tunnel: [_ w153] -> w149
              tunnel: w148 -> [_ w156]
              tunnel: w147 -> [_ w154]
              frame False {
              }
              frame True {
                n140 = call "Enqueue.vi"("Message Data"=w154, "Message"="ReadAcq", "MessageQueue"=w156) -> ("error out"=w153:errorcluster)  [unwired: 7 in, 1 out]
              }
            }
          }
          event User Event {
            n141 = event-data() -> ("ModuleID"=w161:i32, "Data"=w157:variant)  [unwired: 1 in]
            n142 = call <userlib>:"AddressedToThisModule.vi"("ModuleID"=w161, "ModuleAdmin"=w162) -> ("AddressedToThisInstance?"=w160:bool)  [unwired: 8 in, 1 out]
            n143 = case shown="True" w160 {
              tunnel: [_ w163] -> w159
              tunnel: w158 -> [_ w166]
              tunnel: w157 -> [_ w164]
              frame False {
              }
              frame True {
                n144 = call "Enqueue.vi"("Message Data"=w164, "Message"="WriteAcq", "MessageQueue"=w166) -> ("error out"=w163:errorcluster)  [unwired: 7 in, 1 out]
              }
            }
          }
          event User Event {
            n145 = event-data() -> ("ModuleID"=w171:i32, "Data"=w167:variant)  [unwired: 1 in]
            n146 = call <userlib>:"AddressedToThisModule.vi"("ModuleID"=w171, "ModuleAdmin"=w172) -> ("AddressedToThisInstance?"=w170:bool)  [unwired: 8 in, 1 out]
            n147 = case shown="True" w170 {
              tunnel: [_ w173] -> w169
              tunnel: w168 -> [_ w176]
              tunnel: w167 -> [_ w174]
              frame False {
              }
              frame True {
                n148 = call "Enqueue.vi"("Message Data"=w174, "Message"="ConfigAcq", "MessageQueue"=w176) -> ("error out"=w173:errorcluster)  [unwired: 7 in, 1 out]
              }
            }
          }
          event User Event {
            n149 = event-data() -> ("ModuleID"=w181:i32, "Data"=w177:variant)  [unwired: 1 in]
            n150 = call <userlib>:"AddressedToThisModule.vi"("ModuleID"=w181, "ModuleAdmin"=w182) -> ("AddressedToThisInstance?"=w180:bool)  [unwired: 8 in, 1 out]
            n151 = case shown="True" w180 {
              tunnel: [_ w183] -> w179
              tunnel: w178 -> [_ w186]
              tunnel: w177 -> [_ w184]
              frame False {
              }
              frame True {
                n152 = call "Enqueue.vi"("Message Data"=w184, "Message"="ReadTriggers", "MessageQueue"=w186) -> ("error out"=w183:errorcluster)  [unwired: 7 in, 1 out]
              }
            }
          }
          event User Event {
            n153 = event-data() -> ("ModuleID"=w191:i32, "Data"=w187:variant)  [unwired: 1 in]
            n154 = call <userlib>:"AddressedToThisModule.vi"("ModuleID"=w191, "ModuleAdmin"=w192) -> ("AddressedToThisInstance?"=w190:bool)  [unwired: 8 in, 1 out]
            n155 = case shown="True" w190 {
              tunnel: [_ w193] -> w189
              tunnel: w188 -> [_ w196]
              tunnel: w187 -> [_ w194]
              frame False {
              }
              frame True {
                n156 = call "Enqueue.vi"("Message Data"=w194, "Message"="WriteTrigger", "MessageQueue"=w196) -> ("error out"=w193:errorcluster)  [unwired: 7 in, 1 out]
              }
            }
          }
          event User Event {
            n157 = event-data() -> ("ModuleID"=w201:i32, "Data"=w197:variant)  [unwired: 1 in]
            n158 = call <userlib>:"AddressedToThisModule.vi"("ModuleID"=w201, "ModuleAdmin"=w202) -> ("AddressedToThisInstance?"=w200:bool)  [unwired: 8 in, 1 out]
            n159 = case shown="True" w200 {
              tunnel: [_ w203] -> w199
              tunnel: w198 -> [_ w206]
              tunnel: w197 -> [_ w204]
              frame False {
              }
              frame True {
                n160 = call "Enqueue.vi"("Message Data"=w204, "Message"="SyncInfo", "MessageQueue"=w206) -> ("error out"=w203:errorcluster)  [unwired: 7 in, 1 out]
              }
            }
          }
          event User Event {
            n161 = event-data() -> ("ModuleID"=w211:i32, "Data"=w207:variant)  [unwired: 1 in]
            n162 = call <userlib>:"AddressedToThisModule.vi"("ModuleID"=w211, "ModuleAdmin"=w212) -> ("AddressedToThisInstance?"=w210:bool)  [unwired: 8 in, 1 out]
            n163 = case shown="True" w210 {
              tunnel: [_ w213] -> w209
              tunnel: w208 -> [_ w216]
              tunnel: w207 -> [_ w214]
              frame False {
              }
              frame True {
                n164 = call "Enqueue.vi"("Message Data"=w214, "Message"="ConfigTrigger", "MessageQueue"=w216) -> ("error out"=w213:errorcluster)  [unwired: 7 in, 1 out]
              }
            }
          }
          event User Event {
            n165 = event-data() -> ("ModuleID"=w221:i32, "Data"=w217:variant)  [unwired: 1 in]
            n166 = call <userlib>:"AddressedToThisModule.vi"("ModuleID"=w221, "ModuleAdmin"=w222) -> ("AddressedToThisInstance?"=w220:bool)  [unwired: 8 in, 1 out]
            n167 = case shown="True" w220 {
              tunnel: [_ w223] -> w219
              tunnel: w218 -> [_ w226]
              tunnel: w217 -> [_ w224]
              frame False {
              }
              frame True {
                n168 = call "Enqueue.vi"("Message Data"=w224, "Message"="InitDevice", "MessageQueue"=w226) -> ("error out"=w223:errorcluster)  [unwired: 7 in, 1 out]
              }
            }
          }
          event User Event {
            n169 = event-data() -> ("ModuleID"=w231:i32, "Data"=w227:variant)  [unwired: 1 in]
            n170 = call <userlib>:"AddressedToThisModule.vi"("ModuleID"=w231, "ModuleAdmin"=w232) -> ("AddressedToThisInstance?"=w230:bool)  [unwired: 8 in, 1 out]
            n171 = case shown="True" w230 {
              tunnel: [_ w233] -> w229
              tunnel: w228 -> [_ w236]
              tunnel: w227 -> [_ w234]
              frame False {
              }
              frame True {
                n172 = call "Enqueue.vi"("Message Data"=w234, "Message"="FetchWfrms", "MessageQueue"=w236) -> ("error out"=w233:errorcluster)  [unwired: 7 in, 1 out]
              }
            }
          }
          event User Event {
            n173 = event-data() -> ("ModuleID"=w241:i32, "Data"=w237:variant)  [unwired: 1 in]
            n174 = call <userlib>:"AddressedToThisModule.vi"("ModuleID"=w241, "ModuleAdmin"=w242) -> ("AddressedToThisInstance?"=w240:bool)  [unwired: 8 in, 1 out]
            n175 = case shown="True" w240 {
              tunnel: [_ w243] -> w239
              tunnel: w238 -> [_ w246]
              tunnel: w237 -> [_ w244]
              frame False {
              }
              frame True {
                n176 = call "Enqueue.vi"("Message Data"=w244, "Message"="ReadWfrms", "MessageQueue"=w246) -> ("error out"=w243:errorcluster)  [unwired: 7 in, 1 out]
              }
            }
          }
          event User Event {
            n177 = event-data() -> ("ModuleID"=w251:i32, "Data"=w247:variant)  [unwired: 1 in]
            n178 = call <userlib>:"AddressedToThisModule.vi"("ModuleID"=w251, "ModuleAdmin"=w252) -> ("AddressedToThisInstance?"=w250:bool)  [unwired: 8 in, 1 out]
            n179 = case shown="True" w250 {
              tunnel: [_ w253] -> w249
              tunnel: w248 -> [_ w256]
              tunnel: w247 -> [_ w254]
              frame False {
              }
              frame True {
                n180 = call "Enqueue.vi"("Message Data"=w254, "Message"="Abort", "MessageQueue"=w256) -> ("error out"=w253:errorcluster)  [unwired: 7 in, 1 out]
              }
            }
          }
        }
        n181 = call "ErrorHandler.vi"("error in (no error)"=w41, "MessageQueue"=w39) -> ("error out"=w40:errorcluster)  [unwired: 8 in, 1 out]
      }
    }
    frame Error {
      n182 = property class="ModuleAdmin.lvclass"(reference=w589) -> (reference out=w588:refnum<class "ModuleAdmin.lvclass">, "Accessors:CloneRegRef"=w587:refnum<data-value>, "Accessors:Module ID"=w586:i32)  [unwired: 1 in, 1 out]
      n183 = call <userlib>:"Remove.vi"("Module ID"=w586, "CloneRegRef"=w587) -> ("error out"=w591:errorcluster)  [unwired: 7 in, 2 out]
      n184 = flat-sequence {
        tunnel: w592 -> [w595]
        tunnel: w591 -> [_]
        tunnel: [w593] -> w590
        frame #0 {
          w594 = T9 2 items=["no dialog", "OK message", "continue or stop message", "OK message + warnings", "continue/stop + warnings"] ("type of dialog (OK msg:1)")
          n185 = call <vilib>:"Simple Error Handler.vi"("type of dialog (OK msg:1)"=w594, "error in (no error)"=w595) -> ("error out"=w593:errorcluster)  [unwired: 3 in, 4 out]
        }
      }
    }
  }
  n186 = call "DestroyClone.vi"("error in (no error)"=w15, "Exit via Stop Module Req?"=w11, "Wait for Module to stop?"=w12, "ModuleAdmin"=w13) -> ("error out"=w14:errorcluster, "External Launch"=w10:bool)  [unwired: 5 in, 1 out]
  n187 = Unregister For Events(event registration refnum=w7, error in=w8) -> (error out=w5:errorcluster)
  n188 = Release Queue(queue=w4, force destroy? (F)=FALSE, error in (no error)=w14) -> (error out=w9:errorcluster)  [unwired: 2 out]
  n189 = Merge Errors(w5, w9) -> (w6:errorcluster)
  "error out" <- w6
  n190 = case shown="True" w10 {
    tunnel: w6 -> [_ w597]
    frame False {
    }
    frame True {
      n191 = control-ref of="This VI"() -> (w596:refnum<vi>)
      n192 = case shown="No Error" w597 {
        tunnel: w596 -> [w598 w599]
        frame No Error {
          n193 = invoke class="VI" method="FP.Close"(reference=w598) -> ()  [unwired: 2 in, 3 out]
        }
        frame Error {
          n194 = invoke class="VI" method="FP.Open"(reference=w599, "Activate"=TRUE ("Activate?")) -> ()  [unwired: 3 in, 5 out]
        }
      }
    }
  }
